vi "About D-VASim.vi"() -> ()   [LabVIEW 2014]
panel:
  in  "Close":bool
  # "D-VASim (Dynamic Virtual Analyzer and Simulator) is developed in the Department of Applied Mathematics and Computer Science at Technical University of Denmark.\n\nCurrent version: 1.2\nReleased in October 2016\n\nFor help, please contact:\nHasan Baig (haba@dtu.dk)\nJan Madsen (jama@dtu.dk)"
  # "Current versions: 1.2\nRelease in October 2016"
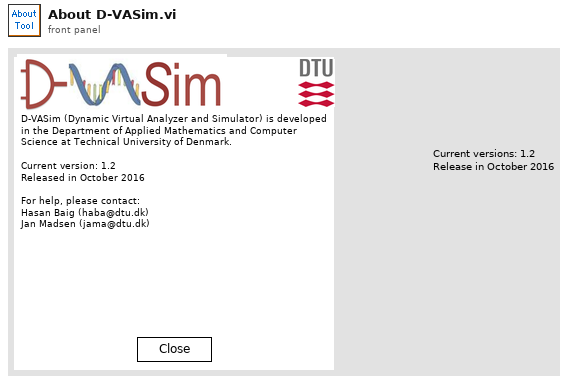
[diagram p1: front panel]
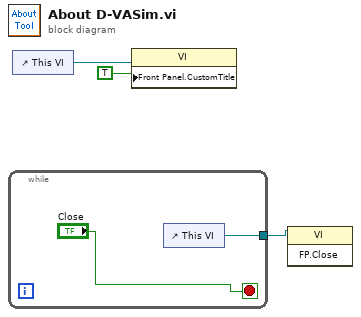
[diagram p0: block diagram]
diagram:
  n1 = while {
    tunnel: [w4] -> w3
    stop <- "Close" stop-if-true
    n2 = control-ref of="This VI"() -> (w4:refnum<vi>)
  }
  n3 = control-ref of="This VI"() -> (w2:refnum<vi>)
  n4 = property class="VI"(reference=w2, "Front Panel.CustomTitle"=TRUE ("Front Panel Window:Custom Title")) -> ()  [unwired: 1 in, 2 out]
  n5 = invoke class="VI" method="FP.Close"(reference=w3) -> ()  [unwired: 2 in, 3 out]
